vi "2_Cross_Correlation.vi"() -> ()   [LabVIEW 2015]
uses:
  C:/Users/MX-Microscope/Documents/LabVIEW Data/lvoop_campus_2018/Detector_Class/Swabian/time_tagger_vis/TTCSharp32.dll
  TTCSharp32.dll
panel:
  out "Cross correlation":cluster{"Y":dbl[], "Y":dbl[]}[](graph)
  # "cross correlation between channels 0 and 1\nbinwidth=1000 ps, n_bins=3000, thus we sample 3000 ns\nwe should see the correlation delta peaks at a bit more than 1000 ns distance"
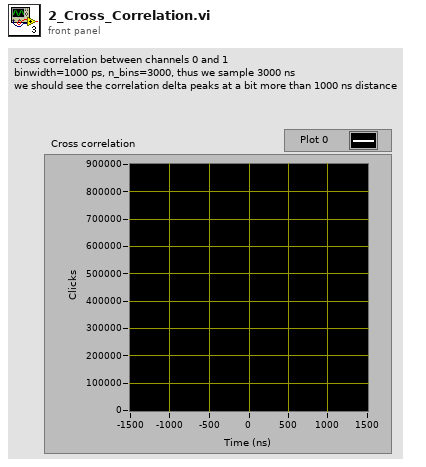
[diagram p1: front panel]
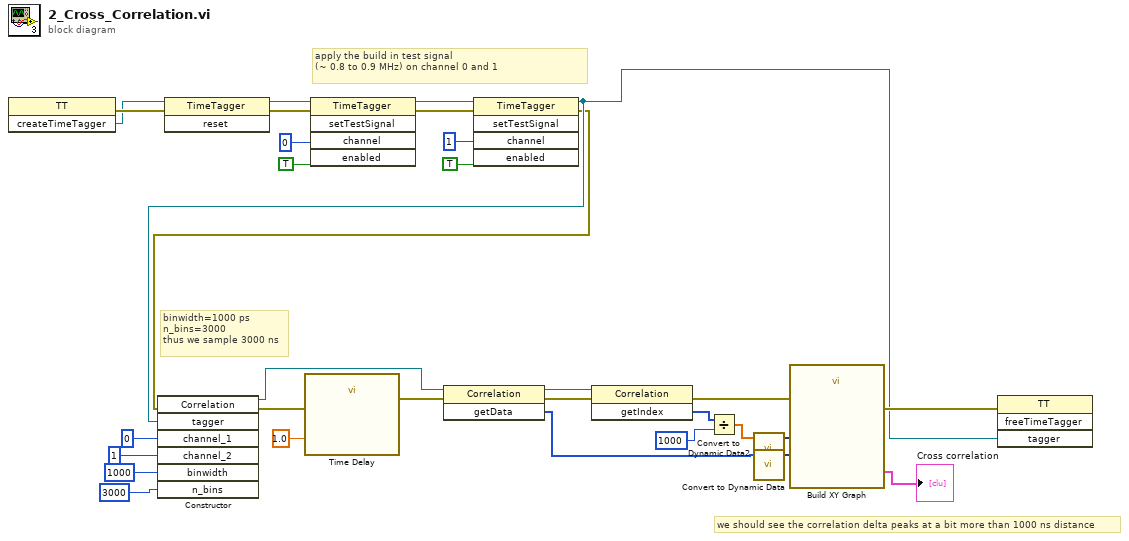
[diagram p0: block diagram]
diagram:
  # "we should see the correlation delta peaks at a bit more than 1000 ns distance"
  # "apply the build in test signal\n(~ 0.8 to 0.9 MHz) on channel 0 and 1"
  # "binwidth=1000 ps\nn_bins=3000\nthus we sample 3000 ns"
  n1 = invoke class="TT" method="createTimeTagger"() -> (error out=w27:errorcluster, "createTimeTagger"=w26:refnum<k24>)  [unwired: 3 in, 1 out]
  n2 = invoke class="TimeTagger" method="reset"(reference=w26, error in=w27) -> (reference out=w14:refnum<k24>, error out=w15:errorcluster)  [unwired: 1 in, 1 out]
  n3 = invoke class="TimeTagger" method="setTestSignal"(reference=w14, error in=w15, "channel"=u32 0, "enabled"=TRUE) -> (reference out=w16:refnum<k24>, error out=w17:errorcluster)  [unwired: 1 in, 3 out]
  n4 = invoke class="TimeTagger" method="setTestSignal"(reference=w16, error in=w17, "channel"=u32 1, "enabled"=TRUE) -> (reference out=w9:refnum<k24>, error out=w6:errorcluster)  [unwired: 1 in, 3 out]
  n5 = constructor class="Correlation"(error in=w6, "tagger"=w9, "channel_1"=u32 0, "channel_2"=u32 1, "binwidth"=i64 1000, "n_bins"=3000) -> (reference out=w5:refnum<k24>, error out=w7:errorcluster)  [unwired: 2 in, 6 out]
  n6 = call "Time Delay"("error in (no error)"=w7, "Delay Time (s)"=1.0) -> ("error out"=w8:errorcluster)  [unwired: 9 in]
  n7 = invoke class="Correlation" method="getData"(reference=w5, error in=w8) -> (reference out=w25:refnum<k24>, error out=w24:errorcluster, "getData"=w1:i32[])  [unwired: 1 in]
  n8 = invoke class="Correlation" method="getIndex"(reference=w25, error in=w24) -> (error out=w22:errorcluster, "getIndex"=w2:i64[])  [unwired: 1 in, 1 out]
  n9 = Divide(x=w2, y=i64 1000) -> (x/y=w3:dbl[])
  n10 = call "Convert to Dynamic Data2"("Array"=w3) -> ("Dynamic Data Type"=w12:dynamicdata)  [unwired: 3 in]
  n11 = call "Convert to Dynamic Data"("Array"=w1) -> ("Dynamic Data Type"=w13:dynamicdata)  [unwired: 3 in]
  n12 = call "Build XY Graph"("error in (no error)"=w22, "Y Input"=w13, "X Input"=w12) -> ("error out"=w10:errorcluster, "XY Graph"=→"Cross correlation":cluster{"X":dbl[], "Y":dbl[]}[])  [unwired: 7 in]
  n13 = invoke class="TT" method="freeTimeTagger"(error in=w10, "tagger"=w9) -> ()  [unwired: 2 in, 4 out]
